vi "App - Push backlog Files to FTP Waiting List.vi"(8 "error in (no error)":errorcluster) -> (0 "error out":errorcluster)   [LabVIEW 2020]
uses:
  Controls/Constants.vi
  Base/Global - FileSync.vi
  Base/Protocol/Protocol.lvclass
  Base/FileSync -- Base.lvlib
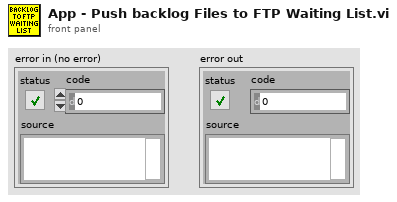
[diagram p1: front panel]
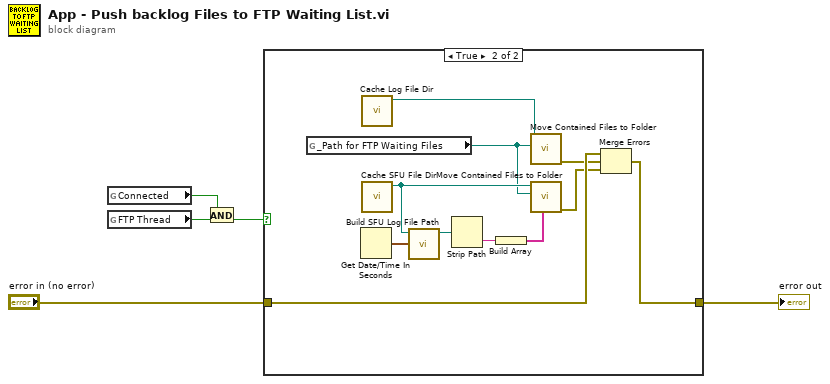
[diagram p0: block diagram]
diagram:
  n1 = global read "Global - FileSync.vi" "Connected"() -> (w1:bool)
  n2 = global read "Constants.vi" "FTP Thread"() -> (w3:bool)
  n3 = And(x=w1, y=w3) -> (x .and. y?=w2:bool)
  n4 = case shown="True" w2 {
    tunnel: [w6 w17] -> w5
    tunnel: "error in (no error)" -> [w6 w16]
    frame False {
    }
    frame True {
      n5 = global read "Constants.vi" "_Path for FTP Waiting Files"() -> (w9:path)
      n6 = Get Date/Time In Seconds() -> (seconds since 1Jan1904=w11:timestamp)
      n7 = call "Cache Log File Dir.vi"() -> ("Cache Log File Dir"=w8:path)  [unwired: 11 in]
      n8 = call "Cache SFU File Dir.vi"() -> ("Cache SFU File Dir"=w10:path)  [unwired: 11 in]
      n9 = call "Build SFU Log File Path.vi"("Time Stamp"=w11, "Log Folder Path"=w10) -> ("appended path"=w12:path)  [unwired: 8 in, 1 out]
      n10 = Strip Path(path=w12) -> (name=w13:string)  [unwired: 1 out]
      n11 = Build Array(w13) -> (w14:string[])
      n12 = call "Move Contained Files to Folder.vi"("Dest Foder Path"=w9, "Folder Path"=w8) -> ("error out"=w7:errorcluster)  [unwired: 9 in]
      n13 = call "Move Contained Files to Folder.vi"("exclued files"=w14, "Dest Foder Path"=w9, "Folder Path"=w10) -> ("error out"=w15:errorcluster)  [unwired: 8 in]
      n14 = Merge Errors(w16, w7, w15) -> (w17:errorcluster)
    }
  }
  "error out" <- w5
